vi "Execute -Polar Plot.vi"(4 "Marking Data":cluster{"magnitude 2":dbl, "phase":dbl}[](array[cluster]), 5 "Display Pic Parameter":T1, 6 "polar attributes":T3, 7 "Plot and scale":T2={"Size Linear plot"=8, "Size point plot"=8, "Plot Scale"=0.0}, 8 "error in (no error)":errorcluster, 9 "Draw Area Size":T4, 10 "data array [mag, phase (deg)]":cluster{"magnitude":dbl, "phase":dbl}[](array[cluster]), 11 "Marking color":u32) -> (0 "error out":errorcluster, 3 "Picture Out":picture)   [LabVIEW 2020]
uses:
  <vilib>/Utility/miscctls.llb/LVBoundsTypeDef.ctl
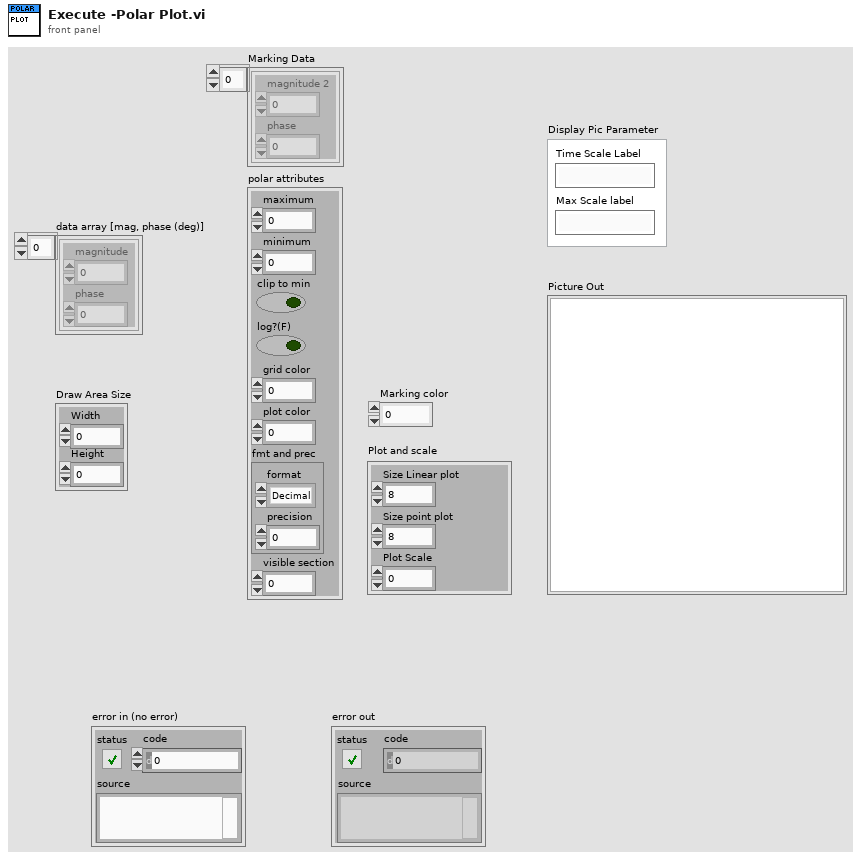
[diagram p1: front panel]
types:
  T1 = cluster{"Time Scale Label":string, "Max Scale label":string}
  T2 = cluster{"Size Linear plot":u16, "Size point plot":u16, "Plot Scale":dbl}
  T3 = cluster{"maximum":dbl, "minimum":dbl, "clip to min":bool, "log?(F)":bool, "grid color":u32, "plot color":u32, "fmt and prec":cluster{"format":enum8{"Decimal", "Scientific", "Engineering", "Binary", "Octal", "Hex"}, "precision":u8}, "visible section":u16}
  T4 = typedef "LVBoundsTypeDef.ctl" = cluster{"Width":u32, "Height":u32}
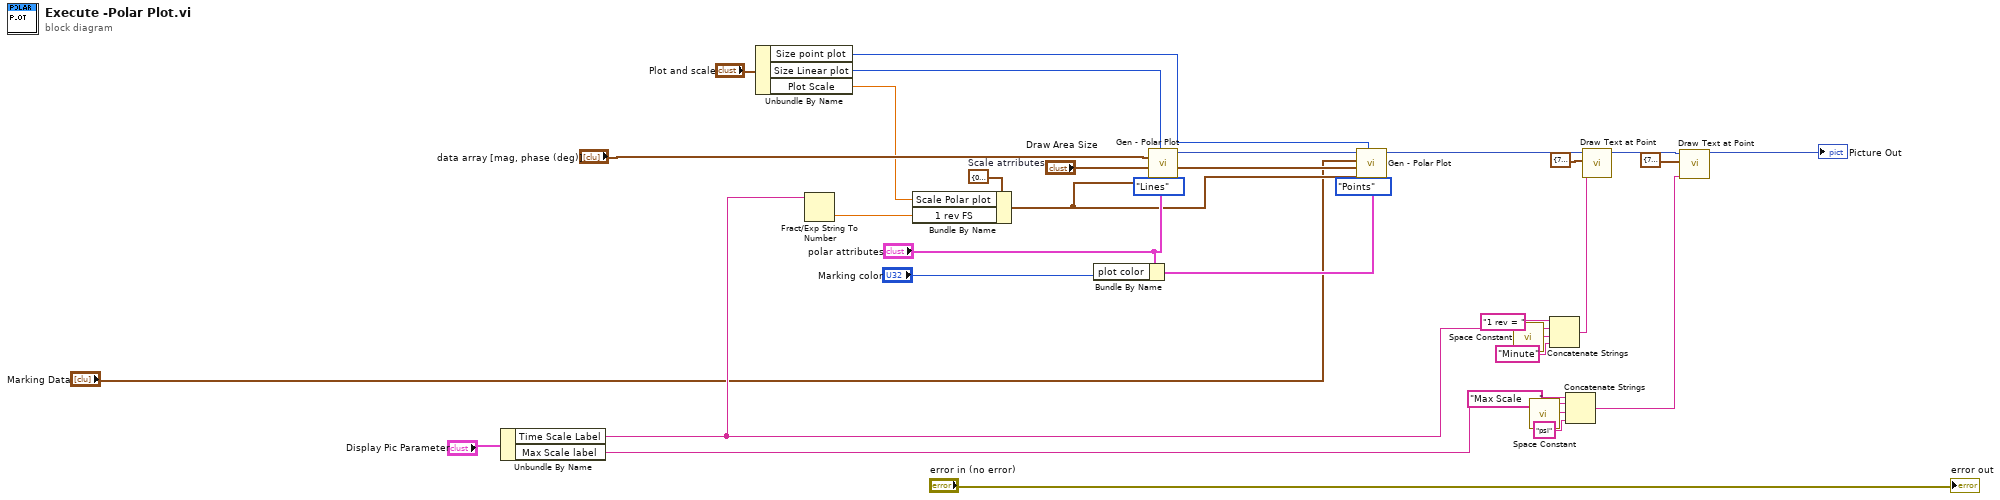
[diagram p0: block diagram]
diagram:
  w5 = cluster{"Scale Polar plot":dbl, "1 rev FS":dbl} {"Scale Polar plot"=0.2, "1 rev FS"=2.0}  # Scale atrributes
  n1 = Unbundle By Name("Display Pic Parameter") -> ("Time Scale Label"=w6:string, "Max Scale label"=w9:string)
  n2 = Unbundle By Name("Plot and scale") -> ("Size point plot"=w25:u16, "Size Linear plot"=w23:u16, "Plot Scale"=w4:dbl)
  n3 = Fract/Exp String To Number(string=w6) -> (number=w1:dbl)  [unwired: 3 in, 1 out]
  n4 = Bundle By Name(cluster=w5, "Scale Polar plot"=w4, "1 rev FS"=w1) -> (w3:cluster{"Scale Polar plot":dbl, "1 rev FS":dbl})
  n5 = Bundle By Name(cluster="polar attributes", "plot color"="Marking color") -> (w30:T3)
  n6 = call "Gen - Polar Plot.vi"("Lines/Points"=enum16{"Lines", "Points"}."Lines", "polar attributes"="polar attributes", "Size"=w23, "Scale atrributes"=w3, "dimensions (w,h)"="Draw Area Size", "data array [mag, phase (deg)]"="data array [mag, phase (deg)]") -> ("new picture"=w29:picture)  [unwired: 5 in]
  n7 = call "Gen - Polar Plot.vi"("Lines/Points"=enum16{"Lines", "Points"}."Points", "polar attributes"=w30, "Size"=w25, "Scale atrributes"=w3, "dimensions (w,h)"="Draw Area Size", "data array [mag, phase (deg)]"="Marking Data", "picture"=w29) -> ("new picture"=w21:picture)  [unwired: 4 in]
  n8 = call <vilib>:"Space Constant.vi"() -> ("String"=w16:string)
  n9 = call <vilib>:"Space Constant.vi"() -> ("String"=w11:string)
  n10 = Concatenate Strings("1 rev = " ("text"), w6, w16, "Minute" ("string")) -> (w19:string)
  n11 = Concatenate Strings("Max Scale  = " ("text"), w9, w11, "psi" ("string")) -> (w7:string)
  n12 = call <vilib>:"Draw Text at Point.vi"("text"=w19, "origin"=cluster{"x":i16, "y":i16} {"x"=722, "y"=35}, "picture"=w21) -> ("new picture"=w14:picture)  [unwired: 7 in, 1 out]
  n13 = call <vilib>:"Draw Text at Point.vi"("text"=w7, "origin"=cluster{"x":i16, "y":i16} {"x"=722, "y"=15}, "picture"=w14) -> ("new picture"=→"Picture Out":picture)  [unwired: 7 in, 1 out]
  "error out" <- "error in (no error)"
